vi "UICtrls_Read_Name_Array.vi"(8 "error in":errorcluster, 10 "Control Label":string[](array[string]), 11 "UI Ref cluster in":T1) -> (0 "error out":errorcluster, 1 "Control Value":variant[](array[variant]), 2 "Found":bool[](array[boolean]), 3 "UI Ref cluster out":T1)   [LabVIEW 2025]
doc: "Read Controls value"
uses:
  UI_Manager/UI_Manager.lvclass
  Controls/UI_Ref_Cluster.ctl
  UI_Manager.lvlib
  <vilib>/Utility/Data Type/Type Definitions/Data Type.ctl
  <vilib>/Utility/Data Type/NI_Data Type.lvlib
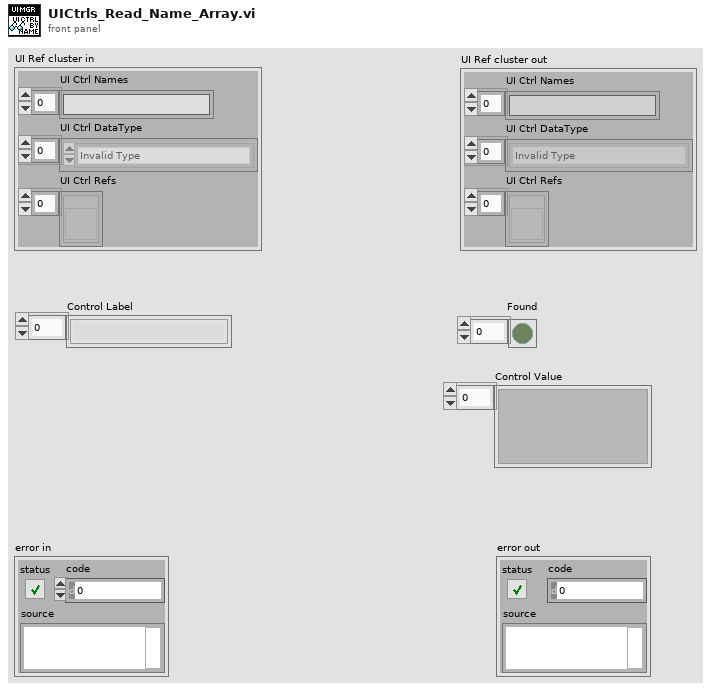
[diagram p1: front panel]
types:
  T1 = typedef "UI_Manager.lvlib/UI_Ref_Cluster.ctl" = cluster{"UI Ctrl Names":string[], "UI Ctrl DataType":T2[], "UI Ctrl Refs":refnum<vi>[]}
  T2 = typedef "NI_Data Type.lvlib/Data Type.ctl" = enum8{"Invalid Type", "Void", "I8", "I16", "I32", "I64", "U8", "U16", "U32", "U64", "Single Float", "Double Float", "Extended Float", "Single Complex", "Double Complex", "Extended Complex", "Enum U8", "Enum U16", "Enum U32", "Enum U64", "Single Float With Unit", "Double Float With Unit", "Extended Float With Unit", "Single Complex with Unit", "Double Complex with Unit", "Extended Complex with Unit", "Boolean", "String", "Path", "Picture", "Tag", "Array", "Cluster", "Variant", "LV Variant", "Waveform", "Timestamp", "Digital Waveform", "Digital Data", "ExpressData", "Refnum", "External Data", "VI", "Poly VI", "LabVIEW Class Instance", "Fixed Point", "Set Collection", "Map Collection"}
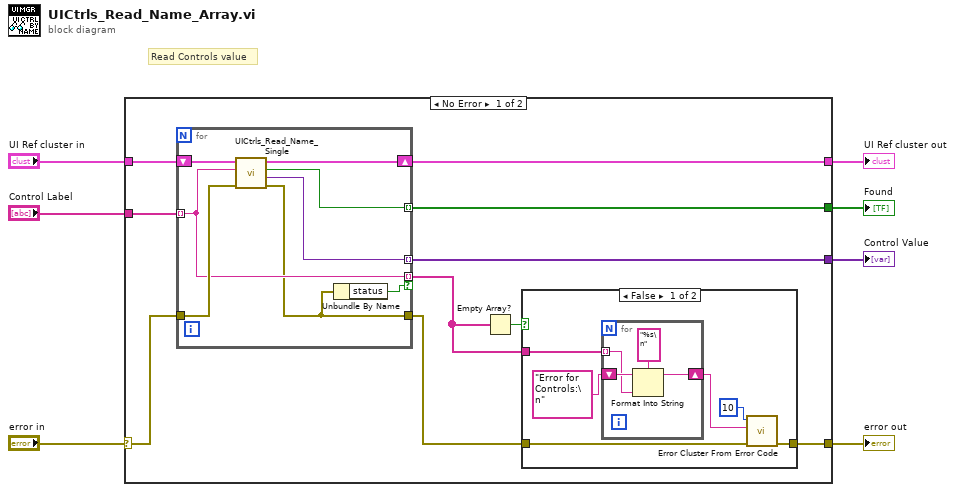
[diagram p0: block diagram]
diagram:
  # "Read Controls value"
  n1 = case shown="No Error" "error in" {
    selector: "error in" -> [w17 w38]
    tunnel: [w10 w38] -> w7
    tunnel: "Control Label" -> [w16 _]
    tunnel: [w14 w37] -> w4
    tunnel: "UI Ref cluster in" -> [w15 w37]
    tunnel: [w12 _] -> w2
    tunnel: [w13 _] -> w1
    frame No Error {
      n2 = for {
        tunnel: w16 -> [w31] mode=indexing
        shift-right: [w34] -> w14
        shift-left: w15 -> [w35]
        tunnel: [w33] -> w13 mode=indexing
        tunnel: [w32] -> w12 mode=indexing
        tunnel: w17 -> [w36]
        tunnel: [w30] -> w9
        tunnel: [w31] -> w8 mode=indexing if=w29
        n3 = call "UICtrls_Read_Name_Single.vi"("error in"=w36, "Control Label"=w31, "UI Ref cluster in"=w35) -> ("error out"=w30:errorcluster, "Control Value"=w32:variant, "Found"=w33:bool, "UI Ref cluster out"=w34:T1)  [unwired: 4 in, 1 out]
        n4 = Unbundle By Name(w30) -> ("status"=w29:bool)
      }
      n5 = Empty Array?(array=w8) -> (empty?=w11:bool)
      n6 = case shown="False" w11 {
        tunnel: [w23 w28] -> w10
        tunnel: w9 -> [w22 w28]
        tunnel: w8 -> [w18 _]
        frame False {
          n7 = for {
            tunnel: w18 -> [w25] mode=indexing
            shift-right: [w27] -> w20
            shift-left: "Error for Controls:\n" -> [w26]
            n8 = Format Into String(format string="%s\n", initial string=w26, w25) -> (resulting string=w27:string)  [unwired: 1 in, 1 out]
          }
          n9 = call <vilib>:"Error Cluster From Error Code.vi"("error in (no error)"=w22, "error message (\"\")"=w20, "error code (0)"=10) -> ("error out"=w23:errorcluster)  [unwired: 6 in]
        }
        frame True {
        }
      }
    }
    frame Error {
    }
  }
  "error out" <- w7
  "Control Value" <- w2
  "UI Ref cluster out" <- w4
  "Found" <- w1
